vi "Test URL.vi"(8 "error in (no error)":errorcluster) -> (0 "error out":errorcluster)   [LabVIEW 2016]
uses:
  Request/Request.lvclass/Request.ctl
  Request/Request.lvclass
  <vilib>/addons/_JKI Toolkits/Caraya/classes/Assert/Assert.lvclass
  <vilib>/addons/_JKI Toolkits/Caraya/classes/Test/Test.lvclass
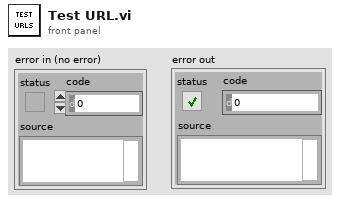
[diagram p1: front panel]
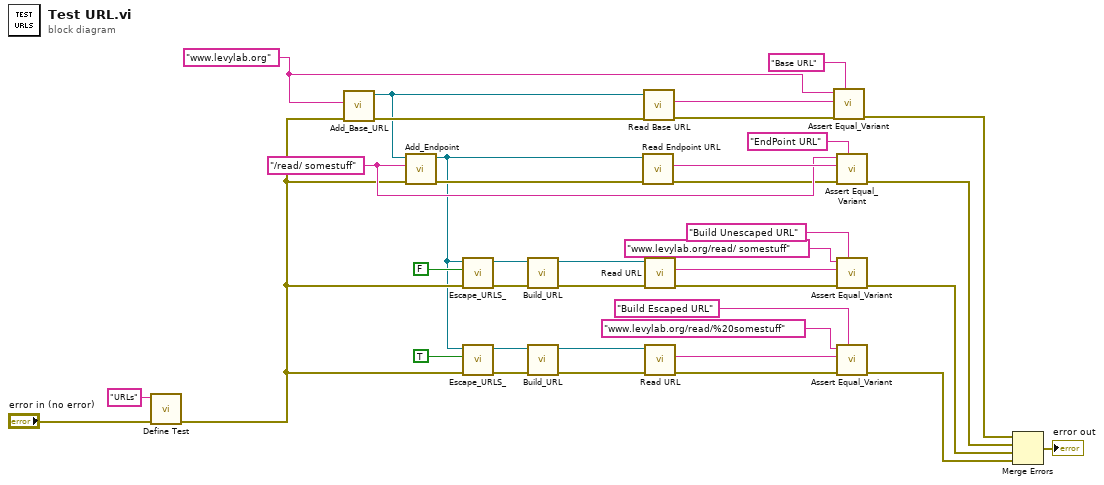
[diagram p0: block diagram]
diagram:
  w30 = "/read/ somestuff" ("Endpoint URL")
  w33 = "www.levylab.org" ("Base URL")
  n1 = call <vilib>:"Define Test.vi"("error in (no error)"="error in (no error)", "Label (VI Title)"="URLs") -> ("error out"=w8:errorcluster)  [unwired: 9 in]
  n2 = call "Add_Base_URL.vi"("error in (no error)"=w8, "Base URL"=w33) -> ("error out"=w36:errorcluster, "Request out"=w32:refnum<class "Request.lvclass">)  [unwired: 8 in]
  n3 = call "Add_Endpoint.vi"("error in (no error)"=w8, "Endpoint URL"=w30, "Request in"=w32) -> ("error out"=w29:errorcluster, "Request out"=w7:refnum<class "Request.lvclass">)  [unwired: 7 in]
  n4 = call "Escape_URLS_.vi"("error in (no error)"=w8, "Escape URLs"=FALSE, "Request in"=w7) -> ("error out"=w18:errorcluster, "Request out"=w19:refnum<class "Request.lvclass">)  [unwired: 7 in]
  n5 = call "Escape_URLS_.vi"("error in (no error)"=w8, "Escape URLs"=TRUE, "Request in"=w7) -> ("error out"=w17:errorcluster, "Request out"=w16:refnum<class "Request.lvclass">)  [unwired: 7 in]
  n6 = call "Build_URL.vi"("error in (no error)"=w18, "Request in"=w19) -> ("error out"=w25:errorcluster, "Request out"=w26:refnum<class "Request.lvclass">)  [unwired: 8 in]
  n7 = call "Build_URL.vi"("error in (no error)"=w17, "Request in"=w16) -> ("error out"=w10:errorcluster, "Request out"=w9:refnum<class "Request.lvclass">)  [unwired: 8 in]
  n8 = call "Read Endpoint URL.vi"("error in (no error)"=w29, "Request in"=w7) -> ("error out"=w28:errorcluster, "Endpoint URL"=w31:string)  [unwired: 7 in, 1 out]
  n9 = call "Read Base URL.vi"("error in (no error)"=w36, "Request in"=w32) -> ("error out"=w37:errorcluster, "Base URL"=w34:string)  [unwired: 7 in, 1 out]
  n10 = call "Read URL.vi"("error in (no error)"=w25, "Request in"=w26) -> ("error out"=w21:errorcluster, "URL"=w24:string)  [unwired: 7 in, 1 out]
  n11 = call "Read URL.vi"("error in (no error)"=w10, "Request in"=w9) -> ("error out"=w14:errorcluster, "URL"=w11:string)  [unwired: 7 in, 1 out]
  n12 = call <vilib>:"Assert Equal_Variant.vi"("Label"="Base URL", "error in (no error)"=w37, "Y"=w34, "X"=w33) -> ("error out"=w5:errorcluster)  [unwired: 7 in]
  n13 = call <vilib>:"Assert Equal_Variant.vi"("Label"="EndPoint URL", "error in (no error)"=w28, "Y"=w31, "X"=w30) -> ("error out"=w4:errorcluster)  [unwired: 7 in]
  n14 = call <vilib>:"Assert Equal_Variant.vi"("Label"="Build Unescaped URL", "error in (no error)"=w21, "Y"=w24, "X"="www.levylab.org/read/ somestuff") -> ("error out"=w3:errorcluster)  [unwired: 7 in]
  n15 = call <vilib>:"Assert Equal_Variant.vi"("Label"="Build Escaped URL", "error in (no error)"=w14, "Y"=w11, "X"="www.levylab.org/read/%20somestuff") -> ("error out"=w2:errorcluster)  [unwired: 7 in]
  n16 = Merge Errors(w5, w4, w3, w2) -> (→"error out":errorcluster)
